vi "PathToMessageMain.vi"(10 "VIName":string, 11 "Service":string) -> (2 "Path":path)   [LabVIEW 2017, in "MessageGen.lvlib"]
uses:
  <vilib>/addons/InsightCM/MessageBus/CodeGen/MessageGen.lvlib
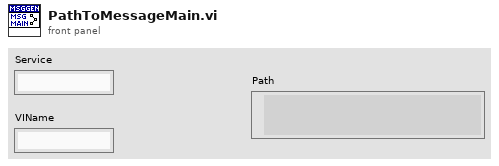
[diagram p1: front panel]
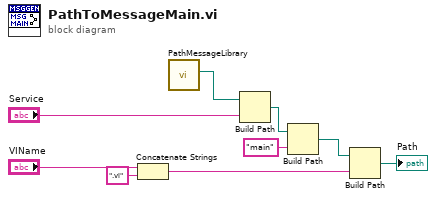
[diagram p0: block diagram]
diagram:
  n1 = Concatenate Strings("VIName", ".vi" ("string")) -> (w2:string)
  n2 = call <vilib>:"PathMessageLibrary.vi"() -> ("Path"=w9:path)  [unwired: 11 in]
  n3 = Build Path(base path=w9, name or relative path="Service") -> (appended path=w4:path)
  n4 = Build Path(base path=w4, name or relative path="main") -> (appended path=w3:path)
  n5 = Build Path(base path=w3, name or relative path=w2) -> (appended path=→"Path":path)
